vi "dscDASetSettings.vi"(8 "error in":errorcluster, 10 "dscDASettings":T1 {"load_cal" items=["FALSE", "TRUE"]}, 11 "board":i16) -> (0 "error out":errorcluster, 2 "dasettings":T1 {"load_cal" items=["FALSE", "TRUE"]}, 3 "boardOut":i16)   [LabVIEW 2011, in "Diamond Universal Driver.lvlib"]
doc: "Set the D/A configuration for future D/A conversions. A delay of approximately 10 us occurs during this function call in order to allow the analog circuit to settle on the new settings. On -AT boards, if <B>load_cal</B> == TRUE, then the calibrations settings are loaded from EEPROM for the current D/A configuration. This results in a slightly more accurate D/A conversion but causes an additional delay of approximately 10 ms."
uses:
  Diamond Universal Driver.lvlib
  Controls/dscDASettings.ctl
  Controls/dscPolarity.ctl
  Controls/dscBool.ctl
  Controls/error codes.ctl
  Instruments/WL OPC/Support/dlls/dscud.dll
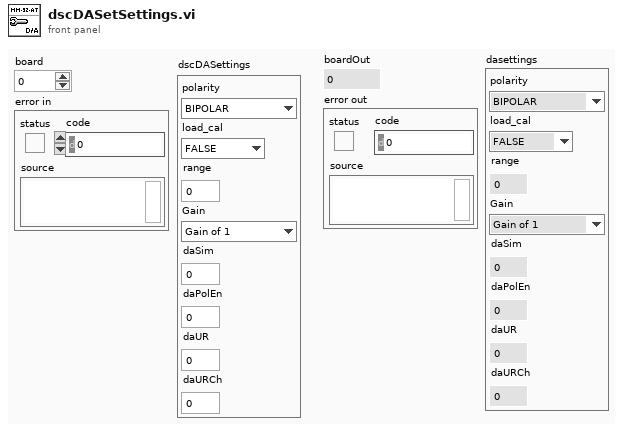
[diagram p1: front panel]
types:
  T1 = typedef "Diamond Universal Driver.lvlib/dscDASettings.ctl" = cluster{"polarity":T2, "load_cal":T3, "range":sgl, "Gain":enum16{"Gain of 1", "Gain of 2", "Gain of 4", "Gain of 8"}, "daSim":u8, "daPolEn":u8, "daUR":u8, "daURCh":u8}
  T2 = typedef "Diamond Universal Driver.lvlib/dscPolarity.ctl" = enum8{"BIPOLAR", "UNIPOLAR"}
  T3 = typedef "dscBool.ctl" = i32
  T4 = typedef "Diamond Universal Driver.lvlib/error codes.ctl" = enum8{"DE_NONE", "DE_HW_FAILURE", "DE_SW_FAILURE", "DE_HW_NOT_SUPPORTED", "DE_SW_NOT_SUPPORTED", "DE_INVALID_PARM", "DE_ALTERNATE_IN_PROGRESS", "DE_NONE_IN_PROGRESS", "DE_BUFFER_ROLLOVER", "DE_INVALID_ERROR_CODE", "DE_ALREADY_PAUSED", "DE_OVERFLOW", "DE_INVALID_FUNC", "DE_DSCUDH_INVALID", "DE_INVALID_BOARD", "DE_BOARD_LIMIT_REACHED", "DE_BOARD_BUSY", "DE_INVALID_WINDRVR_HANDLE", "DE_INVALID_WINDRVR_VERSION", "DE_BAD_WINDRVR_BOARD_INIT", "DE_OPERATION_TIMED_OUT", "DE_INVALID_WINDRVR_KP", "DE_THREAD_FAILURE"}
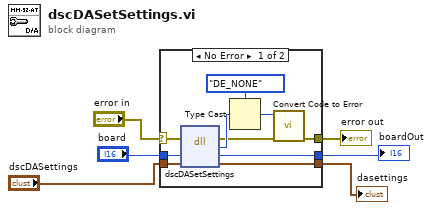
[diagram p0: block diagram]
diagram:
  n1 = case shown="No Error" "error in" {
    selector: "error in" -> [w13 w19]
    tunnel: "board" -> [w11 w18]
    tunnel: [w10 w18] -> w4
    tunnel: [w9 w19] -> w3
    tunnel: "dscDASettings" -> [w8 w17]
    tunnel: [w7 w17] -> w1
    frame No Error {
      n2 = dll-call lib="C:/Users/mrichardson/Documents/Web Based Version Control SW/Instruments/WL OPC/Support/dlls/dscud.dll" fn="dscDASetSettings"(error in=w13, "board"=w11, "dasettings"=w8) -> (error out=w12:errorcluster, "error"=w14:u8, "board"=w10:i16, "dasettings"=w7:T1)  [unwired: 2 in, 1 out]
      n3 = Type Cast(type=error_codes."DE_NONE" ("error codes"), x=w14) -> (*(type *) &x=w16:T4)
      n4 = call "Convert Code to Error.vi"("error in"=w12, "error codes"=w16) -> ("error out"=w9:errorcluster)  [unwired: 9 in]
    }
    frame Error {
    }
  }
  "boardOut" <- w4
  "error out" <- w3
  "dasettings" <- w1
